vi "Relay Command_TS_v2.vi"(8 "error in (no error)":errorcluster, 10 "Relay Command":bool[](array[boolean]), 11 "Control Board VISA":refnum<visa-resource-name>="ControlBoard") -> (0 "error out":errorcluster, 3 "VISA Refnum out":refnum<visa-resource-name>)   [LabVIEW 2022 SP3]
uses:
  <vilib>/Instr/_visa.llb/VISA Flush IO Buffer Mask.ctl
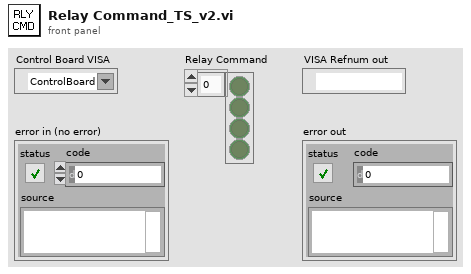
[diagram p1: front panel]
types:
  T1 = typedef "VISA Flush IO Buffer Mask.ctl" = u16
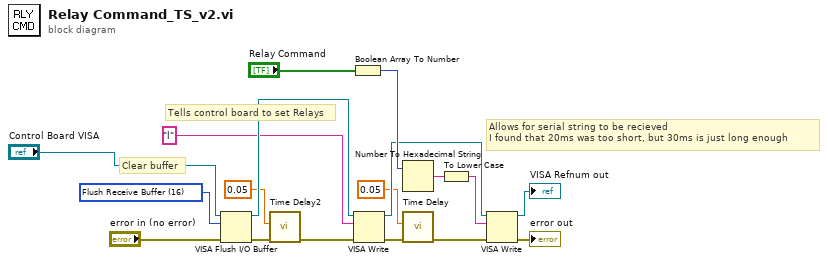
[diagram p0: block diagram]
diagram:
  w12 = T1 16 items=["Flush Receive Buffer"=16, "Write Transmit Buffer to Device"=32, "Flush Receive Buffer (No I/O)"=64, "Flush Transmit Buffer"=128] ("Mask")
  # "Clear buffer"
  # "Allows for serial string to be recieved\nI found that 20ms was too short, but 30ms is just long enough"
  # "Tells control board to set Relays"
  n1 = VISA Flush I/O Buffer(VISA resource name="Control Board VISA", mask (16)=w12, error in (no error)="error in (no error)") -> (VISA resource name out=w17:refnum<visa-resource-name>, error out=w5:errorcluster)
  n2 = call "Time Delay2"("error in (no error)"=w5, "Delay Time (s)"=0.05) -> ("error out"=w4:errorcluster)  [unwired: 9 in]
  n3 = Boolean Array To Number(Boolean array="Relay Command") -> (number=w14:u32)
  n4 = VISA Write(VISA resource name=w17, write buffer="l", error in (no error)=w4) -> (VISA resource name out=w11:refnum<visa-resource-name>, error out=w16:errorcluster)  [unwired: 1 out]
  n5 = Number To Hexadecimal String(2:w14) -> (0:w7:string)  [unwired: 1 in]
  n6 = call "Time Delay"("error in (no error)"=w16, "Delay Time (s)"=0.05) -> ("error out"=w10:errorcluster)  [unwired: 9 in]
  n7 = To Lower Case(string=w7) -> (all lower case string=w6:string)
  n8 = VISA Write(VISA resource name=w11, write buffer=w6, error in (no error)=w10) -> (VISA resource name out=→"VISA Refnum out":refnum<visa-resource-name>, error out=→"error out":errorcluster)  [unwired: 1 out]
